vi "spawned_waitstep.vi"() -> ()   [LabVIEW 2011]
uses:
  <instrlib>/Newport ESP301/Newport ESP301.lvlib
  shared/OnOffTypeDef.ctl
panel:
  in  "output cluster":T2
  in  "VISA resource name":refnum<visa-resource-name>
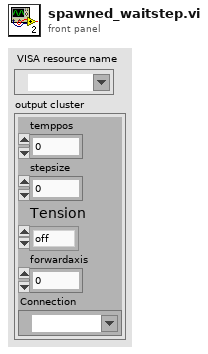
[diagram p1: front panel]
types:
  T1 = typedef "OnOffTypeDef.ctl" = enum16{"off", "on"}
  T2 = cluster{"temppos":dbl, "stepsize":dbl, "Tension":T1, "forwardaxis":i16, "Connection":refnum<visa-resource-name>}
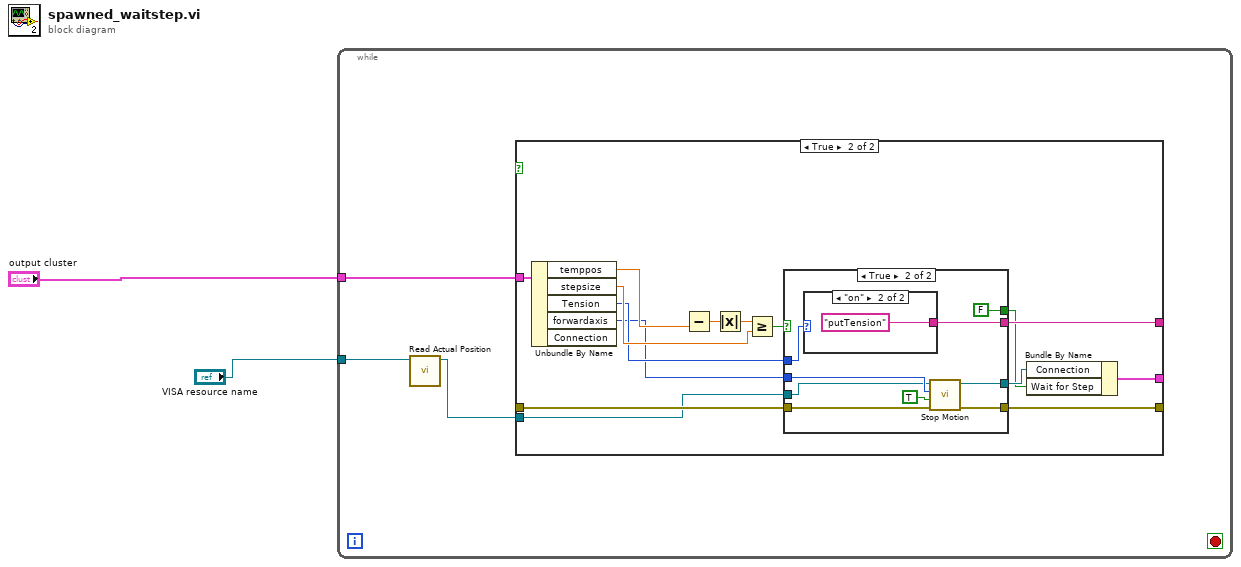
[diagram p0: block diagram]
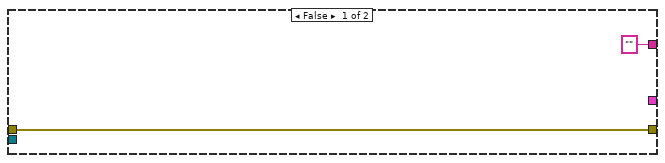
[diagram p2: hidden frame]
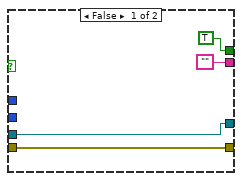
[diagram p3: hidden frame]
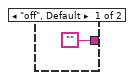
[diagram p4: hidden frame]
diagram:
  n1 = while {
    tunnel: "VISA resource name" -> [w5]
    tunnel: "output cluster" -> [w3]
    stop <- _ stop-if-true
    n2 = call "Read Actual Position.vi"("VISA resource name"=w5) -> ("VISA resource name out"=w4:refnum<visa-resource-name>)  [unwired: 4 in, 2 out]
    n3 = case shown="True" {
      selector: _ -> [_ _]
      tunnel: _ -> [w8 w20]
      tunnel: [w8 w19] -> _
      tunnel: ["" ("new command") w18] -> _
      tunnel: [w6 w17] -> _
      tunnel: w4 -> [_ w14]
      tunnel: w3 -> [_ w13]
      frame False {
      }
      frame True {
        n4 = Unbundle By Name(w13) -> ("temppos"=w12:dbl, "stepsize"=w11:dbl, "Tension"=w10:T1, "forwardaxis"=w9:i16)  [unwired: 1 out]
        n5 = Subtract(y=w12) -> (x-y=w23:dbl)  [unwired: 1 in]
        n6 = Absolute Value(x=w23) -> (abs(x)=w22:dbl)
        n7 = Greater Or Equal?(x=w22, y=w11) -> (x >= y?=w21:bool)
        n8 = case shown="True" w21 {
          tunnel: w10 -> [_ w36]
          tunnel: w9 -> [_ w35]
          tunnel: w14 -> [w27 w34]
          tunnel: w20 -> [w26 w33]
          tunnel: [w26 w32] -> w19
          tunnel: [w27 w30] -> w16
          tunnel: ["" w29] -> w18
          tunnel: [TRUE ("Wait for Step") FALSE ("Wait for Step")] -> w15
          frame False {
          }
          frame True {
            n9 = case shown="\"on\"" w36 {
              tunnel: ["" "putTension"] -> w29
              frame "off", Default {
              }
              frame "on" {
              }
            }
            n10 = call "Stop Motion.vi"("error in (no error)"=w33, "Stop all axes (F)"=TRUE, "Axis (1)"=w35, "VISA resource name"=w34) -> ("error out"=w32:errorcluster, "VISA resource name out"=w30:refnum<visa-resource-name>)  [unwired: 2 in]
          }
        }
        n11 = Bundle By Name("Connection"=w16, "Wait for Step"=w15) -> (w17:cluster{})  [unwired: 1 in]
      }
    }
  }
